vi "Get Empty Cluster.vi"(6 "Name":string, 8 "error in (no error)":errorcluster) -> (0 "error out":errorcluster, 3 "Variant (Cluster) out":variant)   [LabVIEW 2017, in "Advanced Variant Tools.lvlib"]
uses:
  Advanced Variant Tools.lvlib
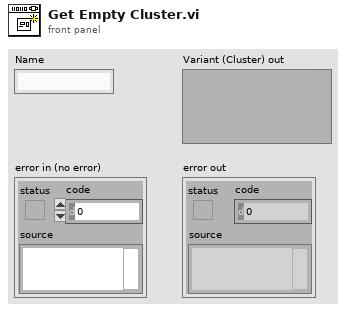
[diagram p1: front panel]
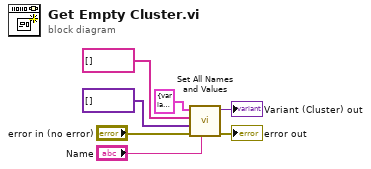
[diagram p0: block diagram]
diagram:
  n1 = call "Set All Names and Values.vi"("Name"="Name", "error in"="error in (no error)", "values"=variant[] [], "Item Names"=string[] [], "Cluster In"=cluster{variant} {variant}) -> ("error out"=→"error out":errorcluster, "Cluster Out"=→"Variant (Cluster) out":variant)  [unwired: 5 in]
